vi "niRFUtil RFHS Channelizer ClearChannelizer CSG.vi"(0 "Channelizer Ref":refnum<data-value>, 11 "error in (no error)":errorcluster) -> (4 "Data Left":csg[](array[numeric]), 6 "Channel Data Len":u32[](array[numeric]), 15 "error out":errorcluster)   [LabVIEW 2015, in "niRFUtil.lvlib"]
uses:
  niRFUtil.lvlib
  Includes/niRFUtil RFHS Channelizer ChannelizerInfo CSG.ctl
  Includes/niRFUtil RFHS Channelizer FilterRef.ctl
  Includes/niRFUtil RFHS Channelizer ChannelizerBufferingMode.ctl
  Utilities/Data FIFO/niRFUtil RFHS FIFO Reference.ctl
  Utilities/Data FIFO/niRFUtil RFHS FIFO.ctl
  Includes/niRFUtil RFHS Channelizer ChannelizerType.ctl
  Includes/niRFUtil RFHS Channelizer ChannelizerFlags.ctl
  Includes/niRFUtil RFHS Channelizer Ref.ctl
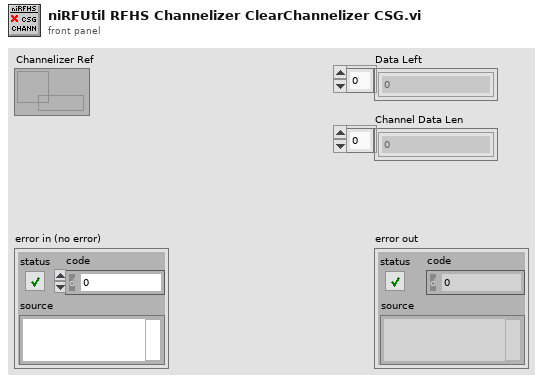
[diagram p1: front panel]
types:
  T1 = typedef "niRFUtil.lvlib/niRFUtil RFHS Channelizer Ref.ctl" = refnum<data-value>
  T2 = typedef "niRFUtil.lvlib/niRFUtil RFHS Channelizer ChannelizerInfo CSG.ctl" = cluster{"Filter LVRef":T3, "Mode":T4, "History":csg[], "Buffer":csg[], "FIFO":T5, "History Len":u32, "Float Cache":csg[], "Double Cache":cdb[], "Type":T7, "Resample Phase":dbl, "fft1Descriptors":u64[], "fft2Descriptors":u64[], "FFT tBuf":csg[], "guardBandLen":i32, "FFT History":csg[], "FFT History Len":u32, "FFTInitDone":u32, "FFT Filter LVRefs":T3[], "FFT fc Offs":u32[], "fft2Sizes":u32[], "BufferW":u32[], "BufferR":u32[], "Buff Off":u32[], "Phase0 (fshift)":dbl[], "Phase (fshift)":dbl[], "fs phase step":dbl[], "Resample Step":dbl, "Flags":T8, "Reset Cnt":i64, "Filter Pass":u32, "Stages":variant[]}
  T3 = typedef "niRFUtil.lvlib/niRFUtil RFHS Channelizer FilterRef.ctl" = cluster{"Ref":u64, "GUID":u64, "Upsample":i32, "Downsample":i32, "Size":i32, "Num Taps":i32}
  T4 = typedef "niRFUtil.lvlib/niRFUtil RFHS Channelizer ChannelizerBufferingMode.ctl" = enum32{"Unbuffered", "Finite", "Continuous"}
  T5 = typedef "niRFUtil.lvlib/niRFUtil RFHS FIFO Reference.ctl" = cluster{"Read Lock":refnum<data-value>, "Info":T6, "Write Lock":refnum<data-value>}
  T6 = typedef "niRFUtil.lvlib/niRFUtil RFHS FIFO.ctl" = cluster{"ID":u64, "Length":u32}
  T7 = typedef "niRFUtil.lvlib/niRFUtil RFHS Channelizer ChannelizerType.ctl" = enum32{"Auto", "Frequency Shift Only", "Resampler Only"}
  T8 = typedef "niRFUtil.lvlib/niRFUtil RFHS Channelizer ChannelizerFlags.ctl" = u32
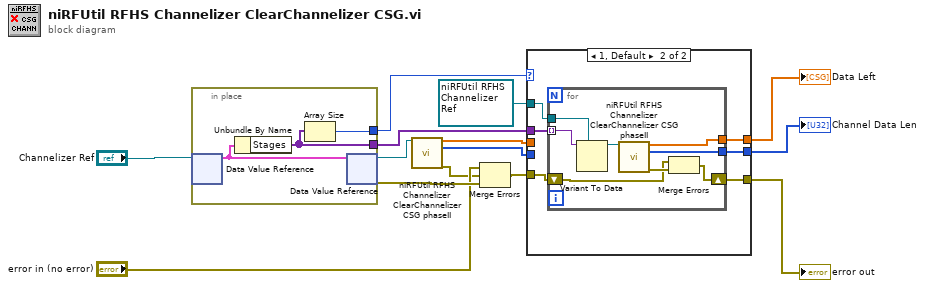
[diagram p0: block diagram]
diagram:
  n1 = in-place {
    in-place-border: [w16] -> w11
    in-place-border: [w15] -> w3
    n2 = in-place-dvr #1("Channelizer Ref") -> (w17:T2)  [unwired: 1 out]
    n3 = Unbundle By Name(w17) -> ("Stages"=w16:variant[])
    n4 = Array Size(array=w16) -> (size(s)=w15:i32)
    n5 = in-place-dvr #1(w17) -> (w12:refnum<data-value>, w13:errorcluster)
  }
  n6 = call "niRFUtil RFHS Channelizer ClearChannelizer CSG phaseII.vi"("Channelizer Ref"=w12) -> ("Data Left"=w5:csg[], "Channel Data Len"=w4:u32[], "error out"=w1:errorcluster)  [unwired: 12 in]
  n7 = Merge Errors("error in (no error)", w1, w13) -> (w7:errorcluster)
  n8 = case shown="1, Default" w3 {
    tunnel: w11 -> [_ w26]
    tunnel: T1 refnum ("Channelizer Ref") -> [_ w25]
    tunnel: [w20 w24] -> w9
    tunnel: [w19 w23] -> w8
    tunnel: w7 -> [w18 w22]
    tunnel: [w18 w21] -> w6
    tunnel: w5 -> [w20 _]
    tunnel: w4 -> [w19 _]
    frame 0 {
    }
    frame 1, Default {
      n9 = for {
        tunnel: w26 -> [w34] mode=indexing
        tunnel: w25 -> [w33]
        tunnel: [w31] -> w24
        tunnel: [w30] -> w23
        shift-right: [w29] -> w21
        shift-left: w22 -> [w27]
        n10 = Variant To Data(type=w33, Variant=w34) -> (data=w32:T1)  [unwired: 1 in, 1 out]
        n11 = call "niRFUtil RFHS Channelizer ClearChannelizer CSG phaseII.vi"("Channelizer Ref"=w32) -> ("Data Left"=w31:csg[], "Channel Data Len"=w30:u32[], "error out"=w28:errorcluster)  [unwired: 12 in]
        n12 = Merge Errors(w27, w28) -> (w29:errorcluster)
      }
    }
  }
  "error out" <- w6
  "Data Left" <- w9
  "Channel Data Len" <- w8
